vi "Destroy_User_Events.vi"(8 "error in (no error)":errorcluster, 11 "Aumentar_contador in":refnum<class "Aumentar_contador.lvclass">) -> (0 "error out":errorcluster, 3 "Aumentar_contador out":refnum<class "Aumentar_contador.lvclass">)   [LabVIEW 2019, in "Aumentar_contador.lvlib" / "Aumentar_contador.lvclass"]
uses:
  Aumentar_contador.lvclass
  Aumentar_contador.lvclass/Aumentar_contador.ctl
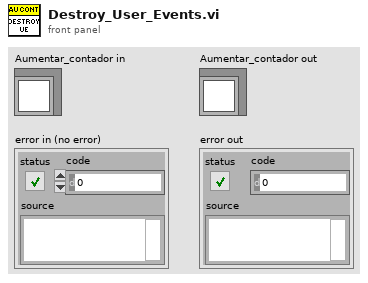
[diagram p1: front panel]
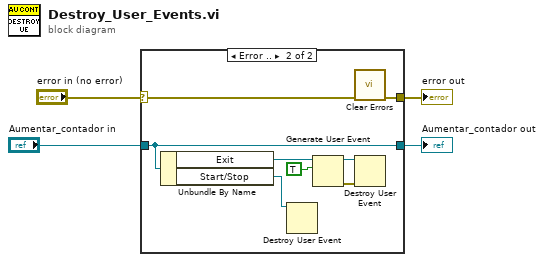
[diagram p0: block diagram]
diagram:
  n1 = case shown="Error .." "error in (no error)" {
    selector: "error in (no error)" -> [w5 w7]
    tunnel: "Aumentar_contador in" -> [w6 w14]
    tunnel: [w6 w14] -> w3
    tunnel: [w5 w8] -> w4
    frame No Error {
    }
    frame Error {
      n2 = Unbundle By Name(w14) -> ("Exit"=w13:refnum<user-event>, "Start/Stop"=w10:refnum<user-event>)
      n3 = Destroy User Event(user event=w10) -> ()  [unwired: 1 in, 1 out]
      n4 = Generate User Event(user event=w13, event data cluster=TRUE ("event data")) -> (user event out=w11:refnum<user-event>, error out=w12:errorcluster)  [unwired: 2 in]
      n5 = call <vilib>:"Clear Errors.vi"("error in (no error)"=w7) -> ("error out"=w8:errorcluster)  [unwired: 5 in, 1 out]
      n6 = Destroy User Event(user event=w11, error in=w12) -> ()  [unwired: 1 out]
    }
  }
  "error out" <- w4
  "Aumentar_contador out" <- w3
